vi "JTAG Power ASIC SPI Test.vi"(11 "error in (no error)":errorcluster) -> (6 "Test Result":string, 15 "error out":errorcluster)   [LabVIEW 2010]
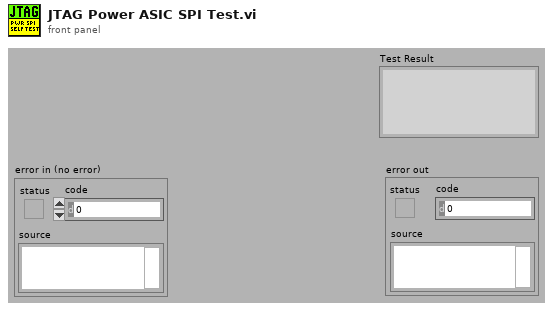
[diagram p1: front panel]
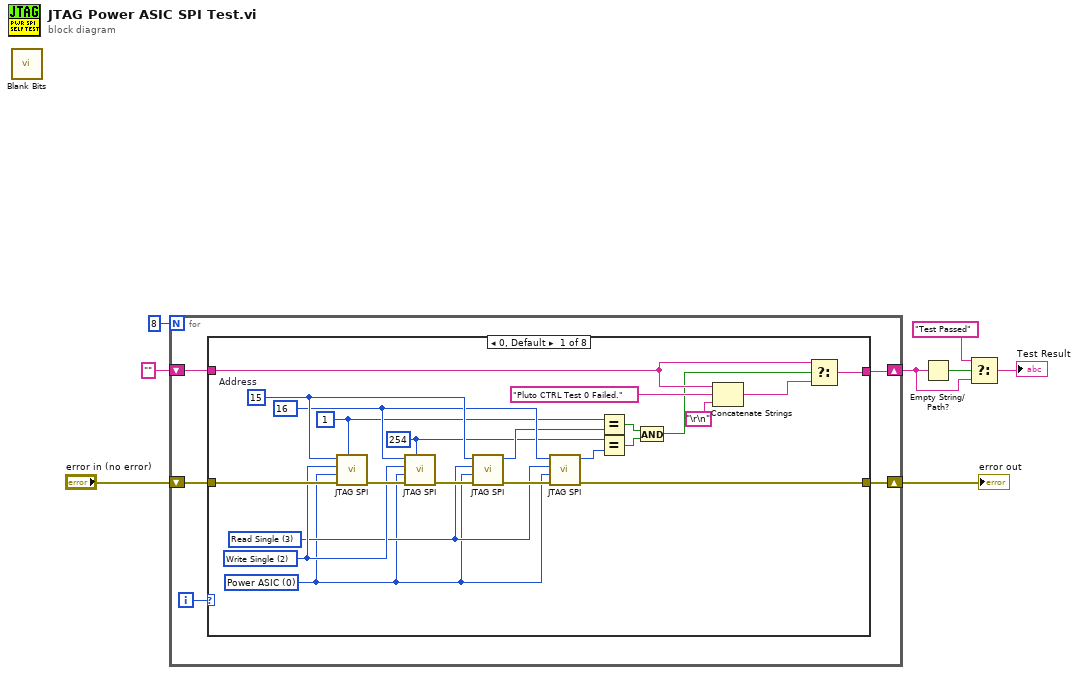
[diagram p0: block diagram]
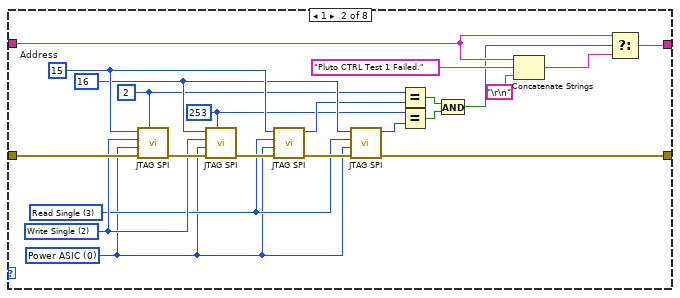
[diagram p2: hidden frame]
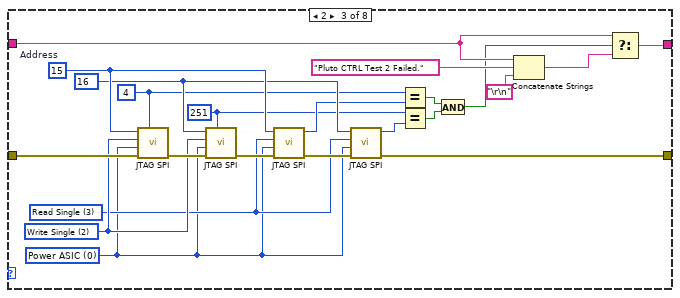
[diagram p3: hidden frame]
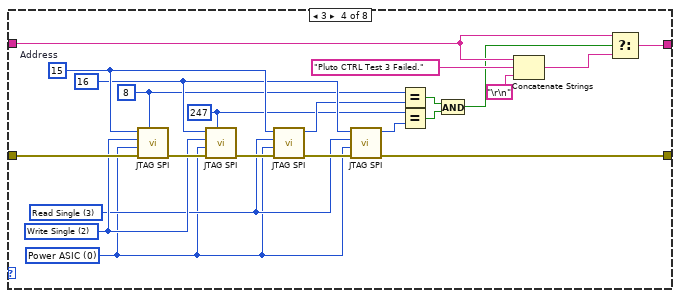
[diagram p4: hidden frame]
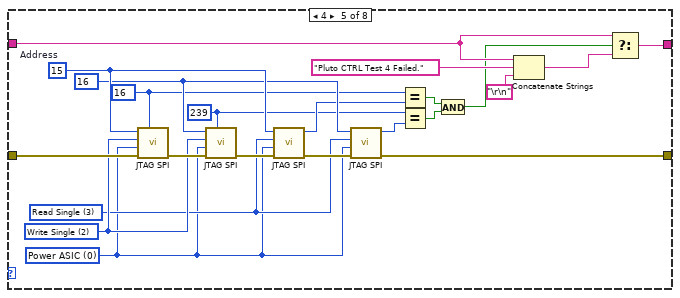
[diagram p5: hidden frame]
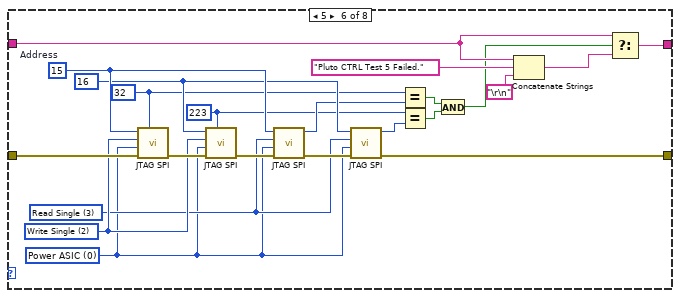
[diagram p6: hidden frame]
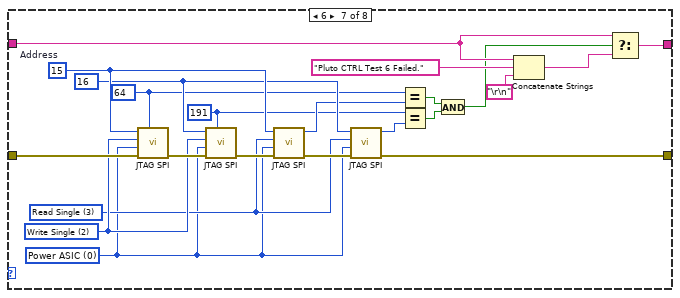
[diagram p7: hidden frame]
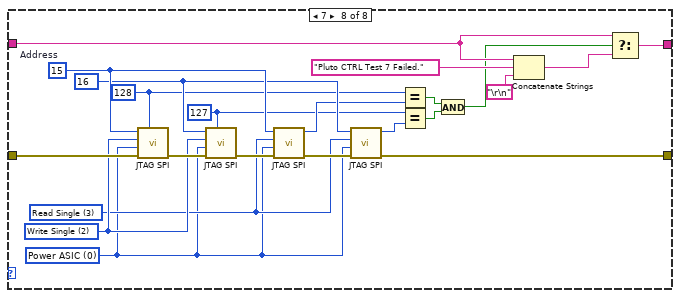
[diagram p8: hidden frame]
diagram:
  n1 = call "Blank Bits.vi"() -> ()  [unwired: 14 in, 2 out]
  n2 = for {
    N: 8 -> [_]
    shift-right: [w12] -> w5
    shift-left: "" -> [w11]
    shift-right: [w10] -> w7
    shift-left: "error in (no error)" -> [w13]
    i -> [w9]
    n3 = case shown="0, Default" w9 {
      tunnel: w13 -> [w35 w57 w79 w101 w123 w145 w167 w189]
      tunnel: [w25 w47 w69 w91 w113 w135 w157 w179] -> w10
      tunnel: [w34 w56 w78 w100 w122 w144 w166 w188] -> w12
      tunnel: w11 -> [w32 w54 w76 w98 w120 w142 w164 w186]
      frame 0, Default {
        w17 = u8 254 ("Value")
        w19 = u8 1 ("Value")
        w21 = u16 3 items=["Power UP", "Power DN", "Write Single", "Read Single", "Write Block", "Read Block", "Write Masked", "Test Value"] ("Function")
        w23 = u16 16 ("Address")
        w20 = u16 0 items=["Power ASIC", "Stim ASIC", "MICS Radio", "FRAM"] ("Target")
        w22 = u16 2 items=["Power UP", "Power DN", "Write Single", "Read Single", "Write Block", "Read Block", "Write Masked", "Test Value"] ("Function")
        w24 = u16 15  # Address
        n4 = call "JTAG SPI.vi"("Value"=w19, "error in (no error)"=w35, "Target"=w20, "Function"=w22, "Address"=w24) -> ("error out"=w28:errorcluster)  [unwired: 3 in, 3 out]
        n5 = call "JTAG SPI.vi"("Value"=w17, "error in (no error)"=w28, "Target"=w20, "Function"=w22, "Address"=w23) -> ("error out"=w27:errorcluster)  [unwired: 3 in, 3 out]
        n6 = call "JTAG SPI.vi"("error in (no error)"=w27, "Target"=w20, "Function"=w21, "Address"=w24) -> ("error out"=w26:errorcluster, "Read Value"=w18:u8)  [unwired: 4 in, 2 out]
        n7 = call "JTAG SPI.vi"("error in (no error)"=w26, "Target"=w20, "Function"=w21, "Address"=w23) -> ("error out"=w25:errorcluster, "Read Value"=w16:u8)  [unwired: 4 in, 2 out]
        n8 = Equal?(x=w19, y=w18) -> (x = y?=w14:bool)
        n9 = Equal?(x=w17, y=w16) -> (x = y?=w33:bool)
        n10 = And(x=w14, y=w33) -> (x .and. y?=w15:bool)
        n11 = Concatenate Strings(w32, "Pluto CTRL Test 0 Failed." ("string"), "\r\n") -> (w31:string)
        n12 = Select(t=w32, s=w15, f=w31) -> (s? t:f=w34:string)
      }
      frame 1 {
        w39 = u8 253 ("Value")
        w41 = u8 2 ("Value")
        w43 = u16 3 items=["Power UP", "Power DN", "Write Single", "Read Single", "Write Block", "Read Block", "Write Masked", "Test Value"] ("Function")
        w45 = u16 16 ("Address")
        w42 = u16 0 items=["Power ASIC", "Stim ASIC", "MICS Radio", "FRAM"] ("Target")
        w44 = u16 2 items=["Power UP", "Power DN", "Write Single", "Read Single", "Write Block", "Read Block", "Write Masked", "Test Value"] ("Function")
        w46 = u16 15  # Address
        n13 = call "JTAG SPI.vi"("Value"=w41, "error in (no error)"=w57, "Target"=w42, "Function"=w44, "Address"=w46) -> ("error out"=w50:errorcluster)  [unwired: 3 in, 3 out]
        n14 = call "JTAG SPI.vi"("Value"=w39, "error in (no error)"=w50, "Target"=w42, "Function"=w44, "Address"=w45) -> ("error out"=w49:errorcluster)  [unwired: 3 in, 3 out]
        n15 = call "JTAG SPI.vi"("error in (no error)"=w49, "Target"=w42, "Function"=w43, "Address"=w46) -> ("error out"=w48:errorcluster, "Read Value"=w40:u8)  [unwired: 4 in, 2 out]
        n16 = call "JTAG SPI.vi"("error in (no error)"=w48, "Target"=w42, "Function"=w43, "Address"=w45) -> ("error out"=w47:errorcluster, "Read Value"=w38:u8)  [unwired: 4 in, 2 out]
        n17 = Equal?(x=w41, y=w40) -> (x = y?=w36:bool)
        n18 = Equal?(x=w39, y=w38) -> (x = y?=w55:bool)
        n19 = And(x=w36, y=w55) -> (x .and. y?=w37:bool)
        n20 = Concatenate Strings(w54, "Pluto CTRL Test 1 Failed." ("string"), "\r\n") -> (w53:string)
        n21 = Select(t=w54, s=w37, f=w53) -> (s? t:f=w56:string)
      }
      frame 2 {
        w61 = u8 251 ("Value")
        w63 = u8 4 ("Value")
        w65 = u16 3 items=["Power UP", "Power DN", "Write Single", "Read Single", "Write Block", "Read Block", "Write Masked", "Test Value"] ("Function")
        w67 = u16 16 ("Address")
        w64 = u16 0 items=["Power ASIC", "Stim ASIC", "MICS Radio", "FRAM"] ("Target")
        w66 = u16 2 items=["Power UP", "Power DN", "Write Single", "Read Single", "Write Block", "Read Block", "Write Masked", "Test Value"] ("Function")
        w68 = u16 15  # Address
        n22 = call "JTAG SPI.vi"("Value"=w63, "error in (no error)"=w79, "Target"=w64, "Function"=w66, "Address"=w68) -> ("error out"=w72:errorcluster)  [unwired: 3 in, 3 out]
        n23 = call "JTAG SPI.vi"("Value"=w61, "error in (no error)"=w72, "Target"=w64, "Function"=w66, "Address"=w67) -> ("error out"=w71:errorcluster)  [unwired: 3 in, 3 out]
        n24 = call "JTAG SPI.vi"("error in (no error)"=w71, "Target"=w64, "Function"=w65, "Address"=w68) -> ("error out"=w70:errorcluster, "Read Value"=w62:u8)  [unwired: 4 in, 2 out]
        n25 = call "JTAG SPI.vi"("error in (no error)"=w70, "Target"=w64, "Function"=w65, "Address"=w67) -> ("error out"=w69:errorcluster, "Read Value"=w60:u8)  [unwired: 4 in, 2 out]
        n26 = Equal?(x=w63, y=w62) -> (x = y?=w58:bool)
        n27 = Equal?(x=w61, y=w60) -> (x = y?=w77:bool)
        n28 = And(x=w58, y=w77) -> (x .and. y?=w59:bool)
        n29 = Concatenate Strings(w76, "Pluto CTRL Test 2 Failed." ("string"), "\r\n") -> (w75:string)
        n30 = Select(t=w76, s=w59, f=w75) -> (s? t:f=w78:string)
      }
      frame 3 {
        w83 = u8 247 ("Value")
        w85 = u8 8 ("Value")
        w87 = u16 3 items=["Power UP", "Power DN", "Write Single", "Read Single", "Write Block", "Read Block", "Write Masked", "Test Value"] ("Function")
        w89 = u16 16 ("Address")
        w86 = u16 0 items=["Power ASIC", "Stim ASIC", "MICS Radio", "FRAM"] ("Target")
        w88 = u16 2 items=["Power UP", "Power DN", "Write Single", "Read Single", "Write Block", "Read Block", "Write Masked", "Test Value"] ("Function")
        w90 = u16 15  # Address
        n31 = call "JTAG SPI.vi"("Value"=w85, "error in (no error)"=w101, "Target"=w86, "Function"=w88, "Address"=w90) -> ("error out"=w94:errorcluster)  [unwired: 3 in, 3 out]
        n32 = call "JTAG SPI.vi"("Value"=w83, "error in (no error)"=w94, "Target"=w86, "Function"=w88, "Address"=w89) -> ("error out"=w93:errorcluster)  [unwired: 3 in, 3 out]
        n33 = call "JTAG SPI.vi"("error in (no error)"=w93, "Target"=w86, "Function"=w87, "Address"=w90) -> ("error out"=w92:errorcluster, "Read Value"=w84:u8)  [unwired: 4 in, 2 out]
        n34 = call "JTAG SPI.vi"("error in (no error)"=w92, "Target"=w86, "Function"=w87, "Address"=w89) -> ("error out"=w91:errorcluster, "Read Value"=w82:u8)  [unwired: 4 in, 2 out]
        n35 = Equal?(x=w85, y=w84) -> (x = y?=w80:bool)
        n36 = Equal?(x=w83, y=w82) -> (x = y?=w99:bool)
        n37 = And(x=w80, y=w99) -> (x .and. y?=w81:bool)
        n38 = Concatenate Strings(w98, "Pluto CTRL Test 3 Failed." ("string"), "\r\n") -> (w97:string)
        n39 = Select(t=w98, s=w81, f=w97) -> (s? t:f=w100:string)
      }
      frame 4 {
        w105 = u8 239 ("Value")
        w107 = u8 16 ("Value")
        w109 = u16 3 items=["Power UP", "Power DN", "Write Single", "Read Single", "Write Block", "Read Block", "Write Masked", "Test Value"] ("Function")
        w111 = u16 16 ("Address")
        w108 = u16 0 items=["Power ASIC", "Stim ASIC", "MICS Radio", "FRAM"] ("Target")
        w110 = u16 2 items=["Power UP", "Power DN", "Write Single", "Read Single", "Write Block", "Read Block", "Write Masked", "Test Value"] ("Function")
        w112 = u16 15  # Address
        n40 = call "JTAG SPI.vi"("Value"=w107, "error in (no error)"=w123, "Target"=w108, "Function"=w110, "Address"=w112) -> ("error out"=w116:errorcluster)  [unwired: 3 in, 3 out]
        n41 = call "JTAG SPI.vi"("Value"=w105, "error in (no error)"=w116, "Target"=w108, "Function"=w110, "Address"=w111) -> ("error out"=w115:errorcluster)  [unwired: 3 in, 3 out]
        n42 = call "JTAG SPI.vi"("error in (no error)"=w115, "Target"=w108, "Function"=w109, "Address"=w112) -> ("error out"=w114:errorcluster, "Read Value"=w106:u8)  [unwired: 4 in, 2 out]
        n43 = call "JTAG SPI.vi"("error in (no error)"=w114, "Target"=w108, "Function"=w109, "Address"=w111) -> ("error out"=w113:errorcluster, "Read Value"=w104:u8)  [unwired: 4 in, 2 out]
        n44 = Equal?(x=w107, y=w106) -> (x = y?=w102:bool)
        n45 = Equal?(x=w105, y=w104) -> (x = y?=w121:bool)
        n46 = And(x=w102, y=w121) -> (x .and. y?=w103:bool)
        n47 = Concatenate Strings(w120, "Pluto CTRL Test 4 Failed." ("string"), "\r\n") -> (w119:string)
        n48 = Select(t=w120, s=w103, f=w119) -> (s? t:f=w122:string)
      }
      frame 5 {
        w127 = u8 223 ("Value")
        w129 = u8 32 ("Value")
        w131 = u16 3 items=["Power UP", "Power DN", "Write Single", "Read Single", "Write Block", "Read Block", "Write Masked", "Test Value"] ("Function")
        w133 = u16 16 ("Address")
        w130 = u16 0 items=["Power ASIC", "Stim ASIC", "MICS Radio", "FRAM"] ("Target")
        w132 = u16 2 items=["Power UP", "Power DN", "Write Single", "Read Single", "Write Block", "Read Block", "Write Masked", "Test Value"] ("Function")
        w134 = u16 15  # Address
        n49 = call "JTAG SPI.vi"("Value"=w129, "error in (no error)"=w145, "Target"=w130, "Function"=w132, "Address"=w134) -> ("error out"=w138:errorcluster)  [unwired: 3 in, 3 out]
        n50 = call "JTAG SPI.vi"("Value"=w127, "error in (no error)"=w138, "Target"=w130, "Function"=w132, "Address"=w133) -> ("error out"=w137:errorcluster)  [unwired: 3 in, 3 out]
        n51 = call "JTAG SPI.vi"("error in (no error)"=w137, "Target"=w130, "Function"=w131, "Address"=w134) -> ("error out"=w136:errorcluster, "Read Value"=w128:u8)  [unwired: 4 in, 2 out]
        n52 = call "JTAG SPI.vi"("error in (no error)"=w136, "Target"=w130, "Function"=w131, "Address"=w133) -> ("error out"=w135:errorcluster, "Read Value"=w126:u8)  [unwired: 4 in, 2 out]
        n53 = Equal?(x=w129, y=w128) -> (x = y?=w124:bool)
        n54 = Equal?(x=w127, y=w126) -> (x = y?=w143:bool)
        n55 = And(x=w124, y=w143) -> (x .and. y?=w125:bool)
        n56 = Concatenate Strings(w142, "Pluto CTRL Test 5 Failed." ("string"), "\r\n") -> (w141:string)
        n57 = Select(t=w142, s=w125, f=w141) -> (s? t:f=w144:string)
      }
      frame 6 {
        w149 = u8 191 ("Value")
        w151 = u8 64 ("Value")
        w153 = u16 3 items=["Power UP", "Power DN", "Write Single", "Read Single", "Write Block", "Read Block", "Write Masked", "Test Value"] ("Function")
        w155 = u16 16 ("Address")
        w152 = u16 0 items=["Power ASIC", "Stim ASIC", "MICS Radio", "FRAM"] ("Target")
        w154 = u16 2 items=["Power UP", "Power DN", "Write Single", "Read Single", "Write Block", "Read Block", "Write Masked", "Test Value"] ("Function")
        w156 = u16 15  # Address
        n58 = call "JTAG SPI.vi"("Value"=w151, "error in (no error)"=w167, "Target"=w152, "Function"=w154, "Address"=w156) -> ("error out"=w160:errorcluster)  [unwired: 3 in, 3 out]
        n59 = call "JTAG SPI.vi"("Value"=w149, "error in (no error)"=w160, "Target"=w152, "Function"=w154, "Address"=w155) -> ("error out"=w159:errorcluster)  [unwired: 3 in, 3 out]
        n60 = call "JTAG SPI.vi"("error in (no error)"=w159, "Target"=w152, "Function"=w153, "Address"=w156) -> ("error out"=w158:errorcluster, "Read Value"=w150:u8)  [unwired: 4 in, 2 out]
        n61 = call "JTAG SPI.vi"("error in (no error)"=w158, "Target"=w152, "Function"=w153, "Address"=w155) -> ("error out"=w157:errorcluster, "Read Value"=w148:u8)  [unwired: 4 in, 2 out]
        n62 = Equal?(x=w151, y=w150) -> (x = y?=w146:bool)
        n63 = Equal?(x=w149, y=w148) -> (x = y?=w165:bool)
        n64 = And(x=w146, y=w165) -> (x .and. y?=w147:bool)
        n65 = Concatenate Strings(w164, "Pluto CTRL Test 6 Failed." ("string"), "\r\n") -> (w163:string)
        n66 = Select(t=w164, s=w147, f=w163) -> (s? t:f=w166:string)
      }
      frame 7 {
        w171 = u8 127 ("Value")
        w173 = u8 128 ("Value")
        w175 = u16 3 items=["Power UP", "Power DN", "Write Single", "Read Single", "Write Block", "Read Block", "Write Masked", "Test Value"] ("Function")
        w177 = u16 16 ("Address")
        w174 = u16 0 items=["Power ASIC", "Stim ASIC", "MICS Radio", "FRAM"] ("Target")
        w176 = u16 2 items=["Power UP", "Power DN", "Write Single", "Read Single", "Write Block", "Read Block", "Write Masked", "Test Value"] ("Function")
        w178 = u16 15  # Address
        n67 = call "JTAG SPI.vi"("Value"=w173, "error in (no error)"=w189, "Target"=w174, "Function"=w176, "Address"=w178) -> ("error out"=w182:errorcluster)  [unwired: 3 in, 3 out]
        n68 = call "JTAG SPI.vi"("Value"=w171, "error in (no error)"=w182, "Target"=w174, "Function"=w176, "Address"=w177) -> ("error out"=w181:errorcluster)  [unwired: 3 in, 3 out]
        n69 = call "JTAG SPI.vi"("error in (no error)"=w181, "Target"=w174, "Function"=w175, "Address"=w178) -> ("error out"=w180:errorcluster, "Read Value"=w172:u8)  [unwired: 4 in, 2 out]
        n70 = call "JTAG SPI.vi"("error in (no error)"=w180, "Target"=w174, "Function"=w175, "Address"=w177) -> ("error out"=w179:errorcluster, "Read Value"=w170:u8)  [unwired: 4 in, 2 out]
        n71 = Equal?(x=w173, y=w172) -> (x = y?=w168:bool)
        n72 = Equal?(x=w171, y=w170) -> (x = y?=w187:bool)
        n73 = And(x=w168, y=w187) -> (x .and. y?=w169:bool)
        n74 = Concatenate Strings(w186, "Pluto CTRL Test 7 Failed." ("string"), "\r\n") -> (w185:string)
        n75 = Select(t=w186, s=w169, f=w185) -> (s? t:f=w188:string)
      }
    }
  }
  "error out" <- w7
  n76 = Empty String/Path?(string/path=w5) -> (empty?=w6:bool)
  n77 = Select(t="Test Passed", s=w6, f=w5) -> (s? t:f=→"Test Result":string)
